vi "Abort_NASA_VIs.vi"(8 "error in":errorcluster, 11 "VI_Refs":refnum<vi>[](array[refnum])) -> (0 "error out":errorcluster)   [LabVIEW 2018]
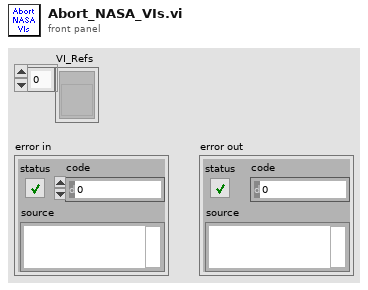
[diagram p1: front panel]
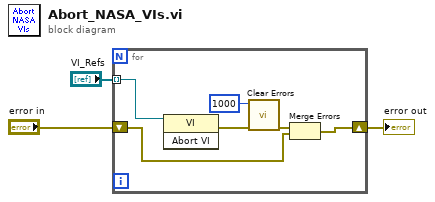
[diagram p0: block diagram]
diagram:
  n1 = for {
    tunnel: "VI_Refs" -> [w9] mode=indexing
    shift-right: [w7] -> w3
    shift-left: "error in" -> [w6]
    n2 = invoke class="VI" method="Abort VI"(reference=w9) -> (error out=w8:errorcluster)  [unwired: 2 in, 2 out]
    n3 = call <vilib>:"Clear Errors.vi"("error in (no error)"=w8, "specific error code to clear (0: all)"=1000) -> ("error out"=w5:errorcluster)  [unwired: 4 in, 1 out]
    n4 = Merge Errors(w5, w6) -> (w7:errorcluster)
  }
  "error out" <- w3
